vi "test.vi"() -> ()   [LabVIEW 2010, in "PointLinkCollection.lvclass"]
uses:
  PointLinkCollection.lvclass
panel:
  in  "buttonSave":bool
  in  "buttonLoad":bool
  in  "buttonStop":bool
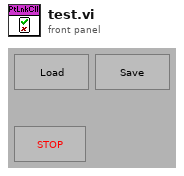
[diagram p1: front panel]
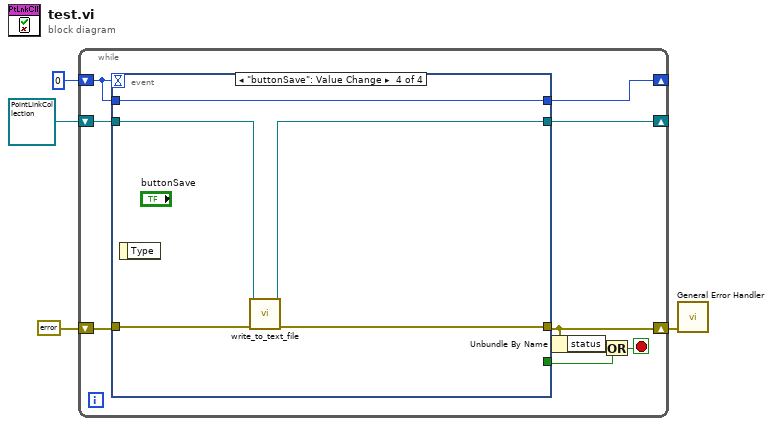
[diagram p0: block diagram]
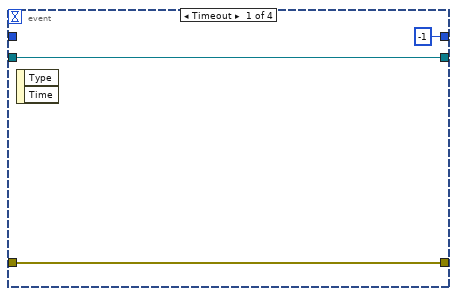
[diagram p2: hidden frame]
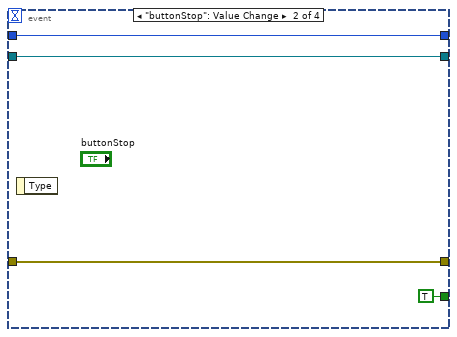
[diagram p3: hidden frame]
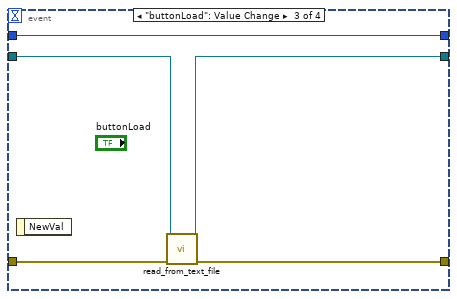
[diagram p4: hidden frame]
diagram:
  n1 = while {
    shift-right: [w12] -> _
    shift-left: 0 -> [w13]
    shift-right: [w10] -> w2
    shift-left: errorcluster {"status"=FALSE, "code"=0, "source"=""} ("error in (no error)") -> [w11]
    shift-right: [w5] -> _
    shift-left: refnum<class "PointLinkCollection.lvclass"> refnum ("PointLinkCollection.lvclass") -> [w6]
    stop <- w7 stop-if-true
    n2 = event shown="[3] \"buttonSave\": Value Change" {
      selector: _ -> [_ _ _ _]
      dyn-events: _ -> [_ _ _ _]
      timeout: w13 -> [_ _ _ _]
      tunnel: [-1 w20 w25 w30] -> w12
      tunnel: w13 -> [_ w20 w25 w30]
      tunnel: [_ TRUE _ _] -> w8
      tunnel: w11 -> [w15 w18 w24 w29]
      tunnel: [w15 w18 w23 w28] -> w10
      tunnel: [w14 w17 w21 w26] -> w5
      tunnel: w6 -> [w14 w17 w22 w27]
      event Timeout {
        n3 = event-data() -> ()  [unwired: 1 in, 2 out]
      }
      event "buttonStop": Value Change {
        n4 = event-data() -> ()  [unwired: 1 in, 1 out]
      }
      event "buttonLoad": Value Change {
        n5 = event-data() -> ()  [unwired: 1 in, 1 out]
        n6 = call "read_from_text_file.vi"("error in (no error)"=w24, "PointLinkCollection in"=w22) -> ("error out"=w23:errorcluster, "PointLinkCollection out"=w21:refnum<class "PointLinkCollection.lvclass">)  [unwired: 8 in]
      }
      event "buttonSave": Value Change {
        n7 = event-data() -> ()  [unwired: 1 in, 1 out]
        n8 = call "write_to_text_file.vi"("error in (no error)"=w29, "PointLinkCollection in"=w27) -> ("error out"=w28:errorcluster, "PointLinkCollection out"=w26:refnum<class "PointLinkCollection.lvclass">)  [unwired: 8 in]
      }
    }
    n9 = Unbundle By Name(w10) -> ("status"=w9:bool)
    n10 = Or(x=w9, y=w8) -> (x .or. y?=w7:bool)
  }
  n11 = call <vilib>:"General Error Handler.vi"("error in (no error)"=w2) -> ()  [unwired: 10 in, 5 out]
